vi "controlAutoReset.vi"(7 "Set":bool, 8 "error in":errorcluster, 9 "enable":bool, 10 "axis in":u8, 11 "connection ID":refnum<k5>) -> (0 "error out":errorcluster, 1 "amplitude [V] out":bool, 2 "axis out":i32, 3 "connection ID":refnum<k5>)   [LabVIEW 2016, in "AMC_VIs.lvlib"]
doc: "This function retrieves or sets whether the position should be reset every time the reference position is detected."
uses:
  AMC_VIs.lvlib
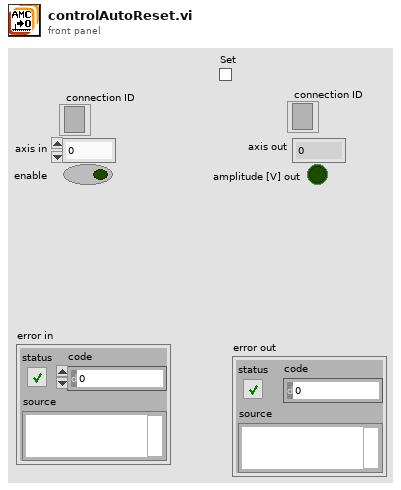
[diagram p1: front panel]
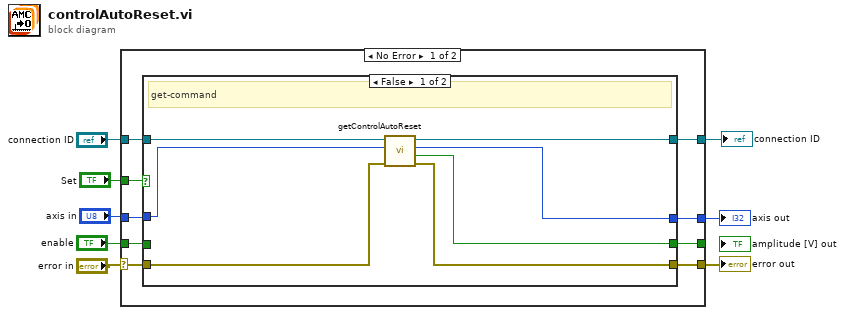
[diagram p0: block diagram]
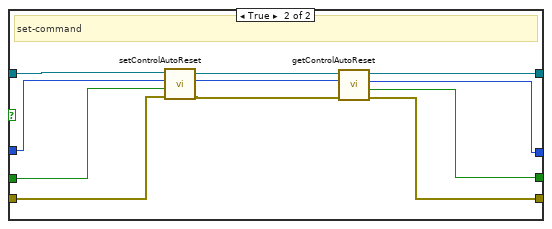
[diagram p2: hidden frame]
diagram:
  n1 = case shown="No Error" "error in" {
    selector: "error in" -> [w12 w39]
    tunnel: "axis in" -> [w17 w37]
    tunnel: [w15 w39] -> w7
    tunnel: "enable" -> [w14 w36]
    tunnel: [w11 w36] -> _
    tunnel: "Set" -> [w13 _]
    tunnel: [w10 w38] -> w5
    tunnel: "connection ID" -> [w16 w38]
    tunnel: [w9 w37] -> w1
    frame No Error {
      n2 = case shown="False" w13 {
        tunnel: w16 -> [w22 w30]
        tunnel: w17 -> [w20 w29]
        tunnel: [w23 w35] -> w15
        tunnel: w14 -> [_ w28]
        tunnel: w12 -> [w24 w34]
        tunnel: [w18 w25] -> w11
        tunnel: [w21 w27] -> w10
        tunnel: [w19 w26] -> w9
        frame False {
          # "get-command"
          n3 = call "getControlAutoReset.vi"("error in"=w24, "axis"=w20, "connection ID"=w22) -> ("error out"=w23:errorcluster, "enabled"=w18:bool, "axis_out"=w19:i32, "connection ID"=w21:refnum<k5>)  [unwired: 5 in]
        }
        frame True {
          # "set-command"
          n4 = call "setControlAutoReset.vi"("error in"=w34, "enable"=w28, "axis"=w29, "connection ID"=w30) -> ("error out"=w33:errorcluster, "axis_out"=w32:i32, "connection ID"=w31:refnum<k5>)  [unwired: 5 in]
          n5 = call "getControlAutoReset.vi"("error in"=w33, "axis"=w32, "connection ID"=w31) -> ("error out"=w35:errorcluster, "enabled"=w25:bool, "axis_out"=w26:i32, "connection ID"=w27:refnum<k5>)  [unwired: 5 in]
        }
      }
    }
    frame Error {
    }
  }
  "error out" <- w7
  "axis out" <- w1
  "connection ID" <- w5
